vi "box catch-national.vi"(9 "vertical":i32, 10 "horizontal":i32) -> (0 "box X":dbl, 1 "pre-height":T1, 2 "height":T1)   [LabVIEW 2019]
uses:
  ctl/height.ctl
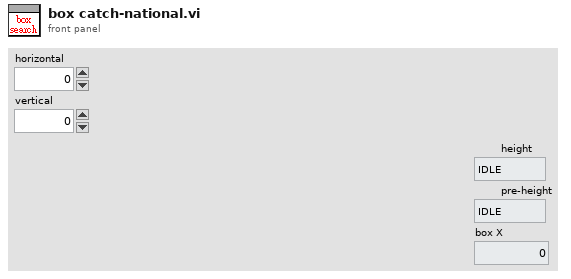
[diagram p1: front panel]
types:
  T1 = typedef "height.ctl" = enum16{"IDLE", "recycle pre-catch", "recycle catch", "recycle zone", "vision height", "box 1", "box 2", "box 3", "box 1 pre", "box 2 pre", "box 3 pre", "reg 1", "reg 2", "reg 1 pre", "reg 2 pre", "put 1", "put 2", "put 3"}
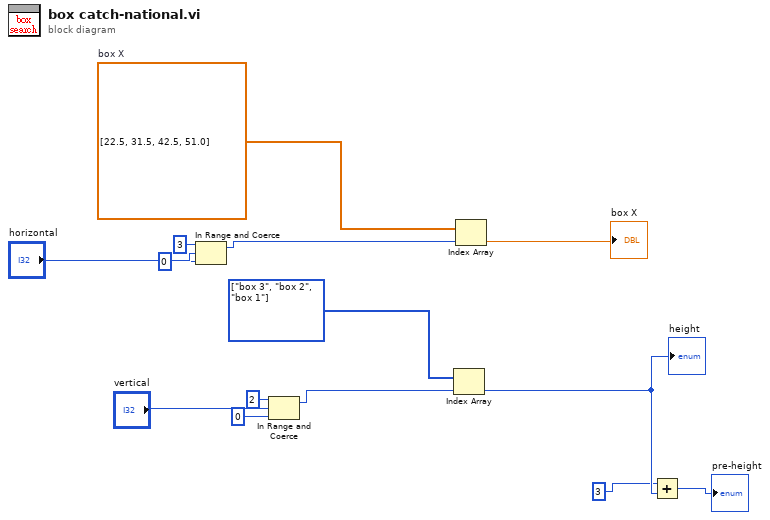
[diagram p0: block diagram]
diagram:
  w14 = T1[] [enum."box 3", enum."box 2", enum."box 1"] items=["IDLE", "recycle pre-catch", "recycle catch", "recycle zone", "vision height", "box 1", "box 2", "box 3", "box 1 pre", "box 2 pre", "box 3 pre", "reg 1", "reg 2", "reg 1 pre", "reg 2 pre", "put 1", "put 2", "put 3"] ("Array")
  w10 = dbl[] [22.5, 31.5, 42.5, 51.0]  # box X
  n1 = In Range and Coerce(upper limit=3, x="horizontal", lower limit=0) -> (coerced(x)=w1:i32)  [unwired: 1 out]
  n2 = In Range and Coerce(upper limit=2, x="vertical", lower limit=0) -> (coerced(x)=w5:i32)  [unwired: 1 out]
  n3 = Index Array(array=w14, index=w5) -> (element=w13:T1)
  "height" <- w13
  n4 = Index Array(array=w10, index=w1) -> (element=→"box X":dbl)
  n5 = Add(x=3, y=w13) -> (x+y=→"pre-height":i32)
